vi "BNO055 receive.vi"(8 "error in (no error)":errorcluster, 11 "rt fifo":refnum<k33>) -> (0 "error out":errorcluster, 3 "rt fifo out":refnum<k33>, 4 "out":dbl)   [LabVIEW 2019]
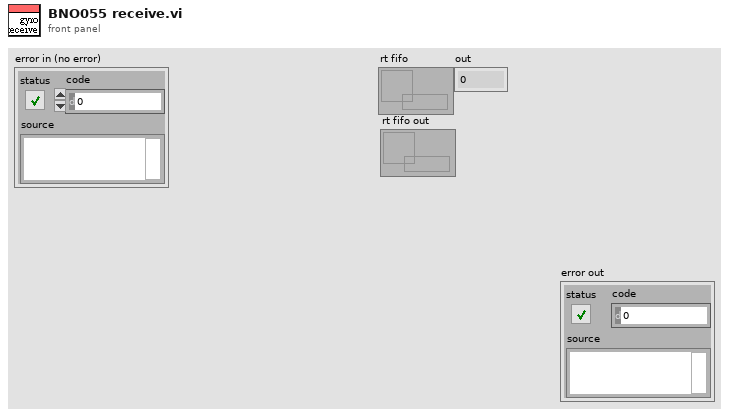
[diagram p1: front panel]
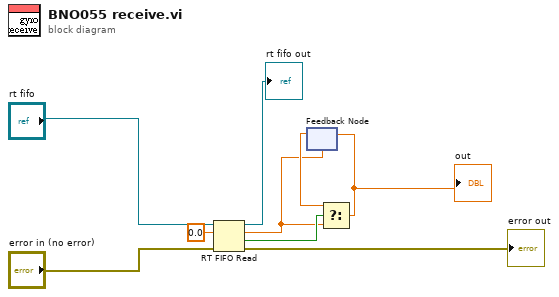
[diagram p0: block diagram]
diagram:
  n1 = RT FIFO Read(0:"rt fifo", 1:0.0 ("element"), 3:"error in (no error)") -> (8:→"rt fifo out":refnum<k33>, 9:w5:dbl, 10:w8:bool, 11:→"error out":errorcluster)  [unwired: 1 in, 1 out]
  n2 = feedback #1(w5) -> (w6:dbl)
  n3 = Select(t=w6, s=w8, f=w5) -> (s? t:f=w7:dbl)
  "out" <- w7
  n4 = feedback-in #1(w7) -> ()
